vi "SW_Load_settings_file.vi"(0 "Controls references":T1) -> (1 "Config file path":path, 2 "error out":errorcluster)   [LabVIEW 2018, in "Tracker.lvlib"]
uses:
  Tracker.lvlib
  <vilib>/Utility/config.llb/NI_LVConfig.lvlib
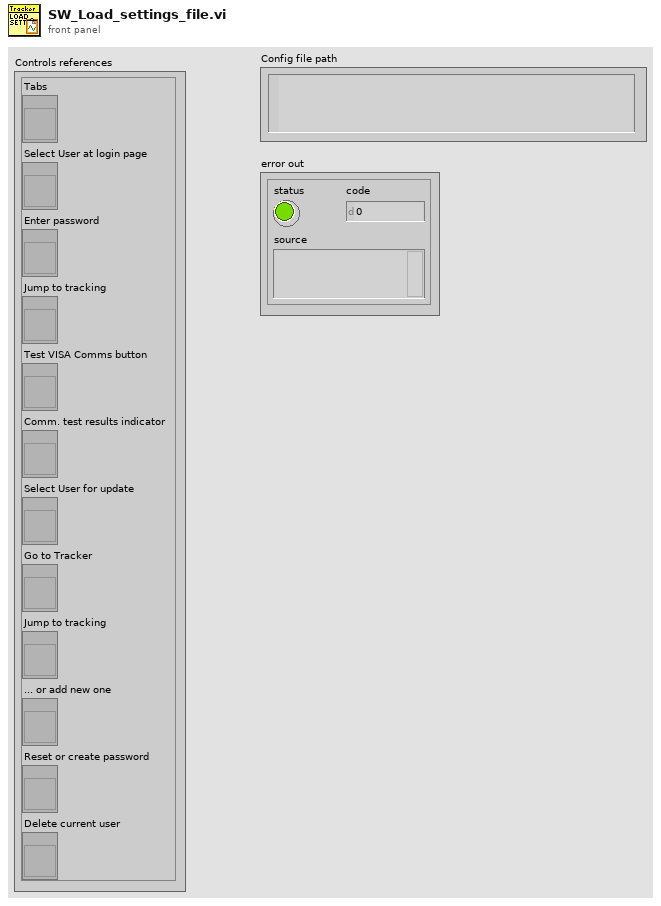
[diagram p1: front panel]
types:
  T1 = cluster{"Tabs":refnum<vi>, "Select User at login page":refnum<vi>, "Enter password":refnum<vi>, "Jump to tracking":refnum<vi>, "Test VISA Comms button":refnum<vi>, "Comm. test results indicator":refnum<vi>, "Select User for update":refnum<vi>, "Go to Tracker":refnum<vi>, "Jump to tracking":refnum<vi>, "... or add new one":refnum<vi>, "Reset or create password":refnum<vi>, "Delete current user":refnum<vi>}
  T2 = enum8{"Enabled", "Disabled", "Disabled and Grayed Out"}
  T3 = enum32{"invalid app kind", "Development System", "Run Time System", "Student Edition", "Embedded LabVIEW", "Evaluation", "Custom"}
  T4 = typedef "NI_LVConfig.lvlib/Config Data RefNum.ctl" = refnum<k1>
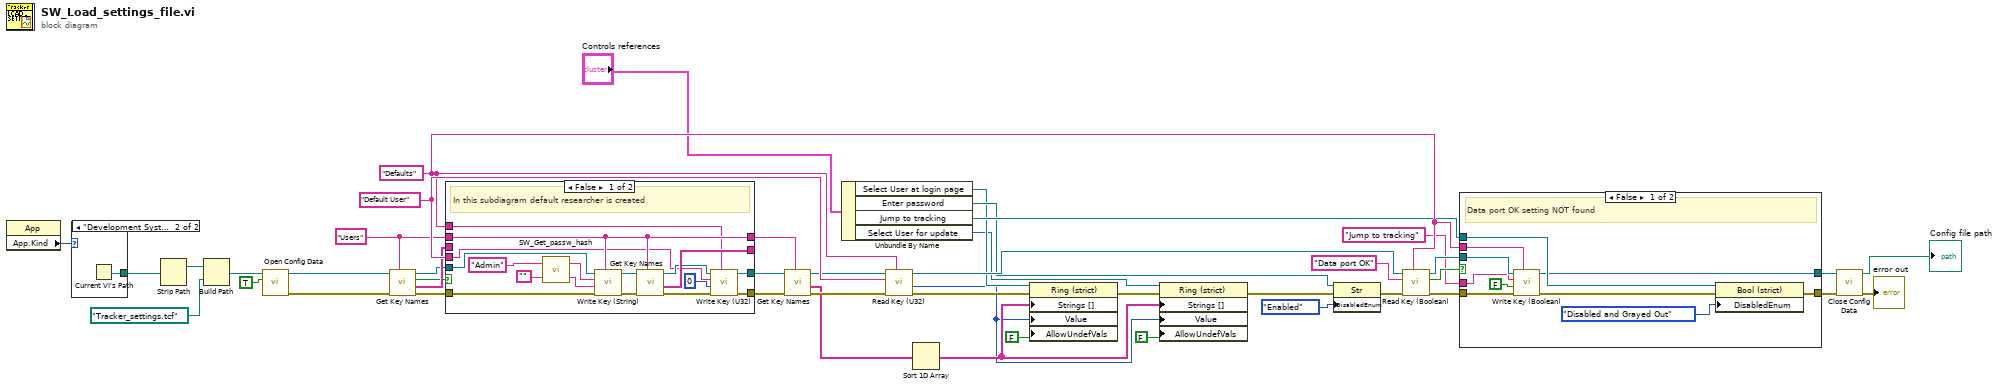
[diagram p0: block diagram]
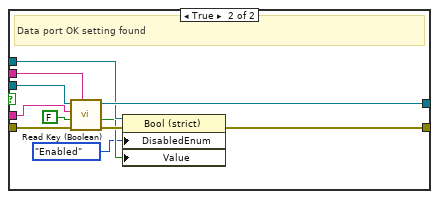
[diagram p2: hidden frame]
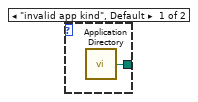
[diagram p4: hidden frame]
diagram:
  w36 = "Users" ("Users section name")
  w41 = "Default User" ("key")
  w21 = "Defaults" ("section")
  n1 = property class="App"() -> ("App.Kind"=w26:T3)  [unwired: 2 in, 2 out]
  n2 = case shown="\"Development System\"" w26 {
    tunnel: [w46 w47] -> w28
    frame "invalid app kind", Default {
      n3 = call <vilib>:"Application Directory.vi"() -> ("Application Directory"=w46:path)
    }
    frame "Development System" {
      n4 = Current VI's Path() -> (path=w47:path)
    }
  }
  n5 = Strip Path(path=w28) -> (stripped path=w29:path)  [unwired: 1 out]
  n6 = Build Path(base path=w29, name or relative path=path "Tracker_settings.tcf") -> (appended path=w15:path)
  n7 = call <vilib>:"Open Config Data.vi"("create file if necessary (T)"=TRUE, "configuration file path"=w15) -> ("error out"=w32:errorcluster, "refnum"=w31:T4)  [unwired: 7 in, 1 out]
  n8 = call <vilib>:"Get Key Names.vi"("section"=w36, "error in (no error)"=w32, "refnum"=w31) -> ("error out"=w34:errorcluster, "key names"=w37:string[], "section exists?"=w33:bool, "refnum out"=w35:T4)  [unwired: 5 in]
  n9 = case shown="False" w33 {
    tunnel: w34 -> [w61 w68]
    tunnel: w35 -> [w62 w67]
    tunnel: w36 -> [w58 w65]
    tunnel: [w52 w67] -> w16
    tunnel: [w53 w68] -> w17
    tunnel: [w63 w66] -> _
    tunnel: w37 -> [_ w66]
    tunnel: [w58 w65] -> w45
    tunnel: w21 -> [w51 _]
    tunnel: w41 -> [w50 _]
    frame False {
      # "In this subdiagram default researcher is created"
      n10 = call "SW_Get_passw_hash.vi"("Password"="" ("string"), "Username"="Admin" ("string")) -> ("Password hash"=w56:string, "Username"=w57:string)
      n11 = call <vilib>:"Write Key (String).vi"("section"=w58, "error in (no error)"=w61, "value"=w56, "key"=w57, "refnum"=w62) -> ("error out"=w60:errorcluster, "refnum out"=w59:T4)  [unwired: 4 in, 1 out]
      n12 = call <vilib>:"Get Key Names.vi"("section"=w58, "error in (no error)"=w60, "refnum"=w59) -> ("error out"=w54:errorcluster, "key names"=w63:string[], "refnum out"=w55:T4)  [unwired: 5 in, 1 out]
      n13 = call <vilib>:"Write Key (U32).vi"("section"=w51, "error in (no error)"=w54, "value"=u32 0, "key"=w50, "refnum"=w55) -> ("error out"=w53:errorcluster, "refnum out"=w52:T4)  [unwired: 4 in, 1 out]
    }
    frame True {
    }
  }
  n14 = call <vilib>:"Get Key Names.vi"("section"=w45, "error in (no error)"=w17, "refnum"=w16) -> ("error out"=w40:errorcluster, "key names"=w38:string[], "refnum out"=w39:T4)  [unwired: 5 in, 1 out]
  n15 = Unbundle By Name("Controls references") -> ("Select User at login page"=w8:refnum<vi>, "Enter password"=w9:refnum<vi>, "Jump to tracking"=w10:refnum<vi>, "Select User for update"=w4:refnum<vi>)
  n16 = call <vilib>:"Read Key (U32).vi"("section"=w21, "error in (no error)"=w40, "key"=w41, "refnum"=w39) -> ("error out"=w42:errorcluster, "value"=w6:u32, "refnum out"=w25:T4)  [unwired: 4 in, 1 out]
  n17 = Sort 1D Array(array=w38) -> (sorted array=w7:string[])
  n18 = property on="Property Node" class="Ring (strict)"(reference=w8, error in=w42, "Strings []"=w7, "Value"=w6, "AllowUndefVals"=FALSE ("Allow Undefined Strings")) -> (error out=w3:errorcluster)  [unwired: 1 out]
  n19 = property on="Property Node" class="Ring (strict)"(reference=w4, error in=w3, "Strings []"=w7, "Value"=w6, "AllowUndefVals"=FALSE ("Allow Undefined Values")) -> (error out=w2:errorcluster)  [unwired: 1 out]
  n20 = property on="Property Node" class="Str"(reference=w9, error in=w2, "DisabledEnum"=T2."Enabled" ("Disabled")) -> (error out=w19:errorcluster)  [unwired: 1 out]
  n21 = call <vilib>:"Read Key (Boolean).vi"("section"=w21, "error in (no error)"=w19, "key"="Data port OK", "refnum"=w25) -> ("error out"=w18:errorcluster, "found?"=w23:bool, "refnum out"=w22:T4)  [unwired: 4 in, 1 out]
  n22 = case shown="False" w23 {
    tunnel: w22 -> [w77 w89]
    tunnel: w21 -> [w74 w88]
    tunnel: [w76 w87] -> w12
    tunnel: w10 -> [w78 w86]
    tunnel: "Jump to tracking" ("key") -> [w75 w85]
    tunnel: w18 -> [w73 w84]
    tunnel: [w71 w82] -> w14
    frame False {
      # "Data port OK setting NOT found"
      n23 = call <vilib>:"Write Key (Boolean).vi"("section"=w74, "error in (no error)"=w73, "value"=FALSE, "key"=w75, "refnum"=w77) -> ("error out"=w72:errorcluster, "refnum out"=w76:T4)  [unwired: 4 in, 1 out]
      n24 = property on="Property Node" class="Bool (strict)"(reference=w78, error in=w72, "DisabledEnum"=T2."Disabled and Grayed Out" ("Disabled")) -> (error out=w71:errorcluster)  [unwired: 1 out]
    }
    frame True {
      # "Data port OK setting found"
      n25 = call <vilib>:"Read Key (Boolean).vi"("section"=w88, "error in (no error)"=w84, "default value"=FALSE, "key"=w85, "refnum"=w89) -> ("error out"=w83:errorcluster, "value"=w80:bool, "refnum out"=w87:T4)  [unwired: 3 in, 1 out]
      n26 = property on="Property Node" class="Bool (strict)"(reference=w86, error in=w83, "DisabledEnum"=T2."Enabled" ("Disabled"), "Value"=w80) -> (error out=w82:errorcluster)  [unwired: 1 out]
    }
  }
  n27 = call <vilib>:"Close Config Data.vi"("error in (no error)"=w14, "refnum"=w12) -> ("error out"=→"error out":errorcluster, "file path"=→"Config file path":path)  [unwired: 8 in]
